vi "GetImage.vi"(0 "XRef":T4, 1 "State In":T3) -> (14 "Image":T2, 15 "Fatal Error Out":T1)   [LabVIEW 2015, in "LVJSON.lvlib" / "Build JSON Array.xnode"]
uses:
  Build JSON Array.xnode
  <vilib>/XNodeSupport/XNodeXNodeRef.ctl
  State.ctl
  <vilib>/XNodeSupport/XNodeImage.ctl
  <vilib>/XNodeSupport/XNodeErrorCluster.ctl
  dimensions.vi
  <vilib>/XNodeSupport/NI_XNodeSupport.lvlib
panel:
  out "image depth 2":i32
  out "image type 2":i32
  out "image depth":i32
  out "image type":i32
  out "size(s) 2":i32
  out "size(s)":i32
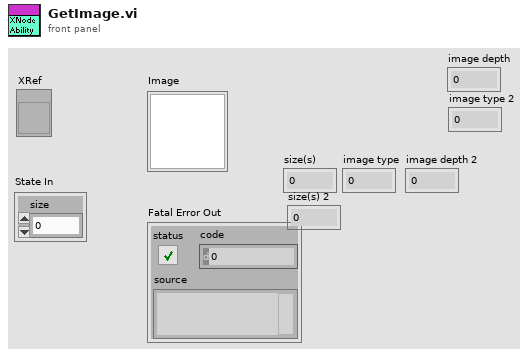
[diagram p1: front panel]
types:
  T1 = typedef "NI_XNodeSupport.lvlib/XNodeErrorCluster.ctl" = errorcluster
  T2 = typedef "NI_XNodeSupport.lvlib/XNodeImage.ctl" = picture
  T3 = typedef "LVJSON.lvlib/Build JSON Array.xnode/State.ctl" = cluster{"size":u32}
  T4 = typedef "NI_XNodeSupport.lvlib/XNodeXNodeRef.ctl" = refnum<vi>
  T5 = typedef "imagedata.ctl" = cluster{"image type":i32, "image depth":i32, "image":u8[], "mask":u8[], "colors":u32[], "Rectangle":cluster{"left":i16, "top":i16, "right":i16, "bottom":i16}}
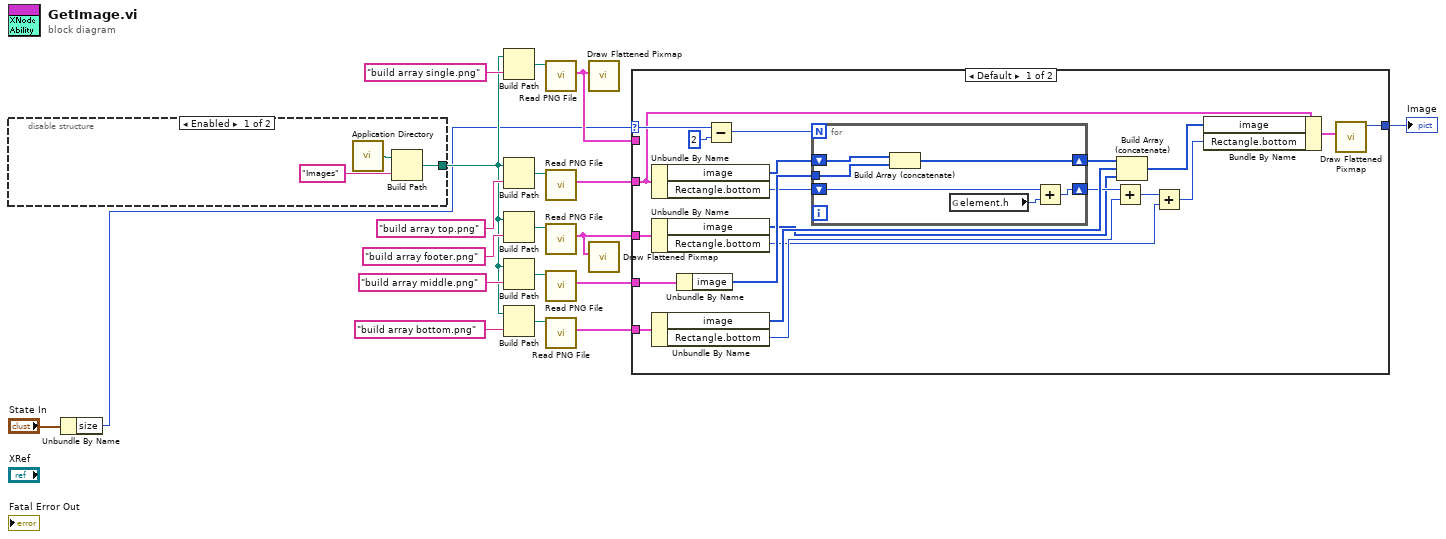
[diagram p0: block diagram]
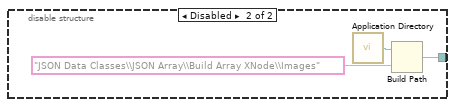
[diagram p2: hidden frame]
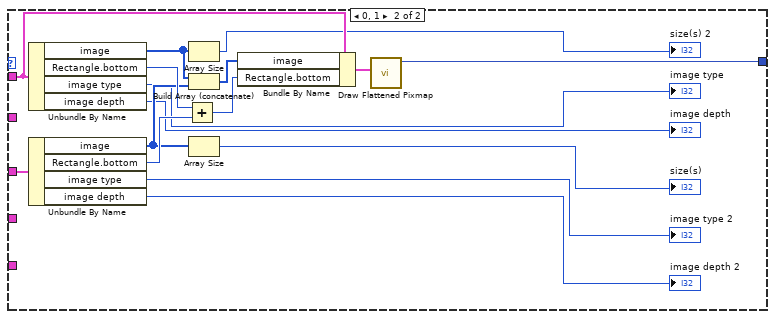
[diagram p3: hidden frame]
diagram:
  n1 = disable-structure shown="Enabled" {
    disable-tunnel: [w21 w24] -> w3
    frame Enabled {
      n2 = call <vilib>:"Application Directory.vi"() -> ("Application Directory"=w20:path)
      n3 = Build Path(base path=w20, name or relative path="Images") -> (appended path=w21:path)
    }
    frame Disabled {
      n4 = call <vilib>:"Application Directory.vi"() -> ("Application Directory"=w23:path)
      n5 = Build Path(base path=w23, name or relative path="JSON Data Classes\\JSON Array\\Build Array XNode\\Images") -> (appended path=w24:path)
    }
  }
  n6 = Unbundle By Name("State In") -> ("size"=w1:u32)
  n7 = Build Path(base path=w3, name or relative path="build array single.png") -> (appended path=w12:path)
  n8 = Build Path(base path=w3, name or relative path="build array top.png") -> (appended path=w9:path)
  n9 = Build Path(base path=w3, name or relative path="build array footer.png") -> (appended path=w5:path)
  n10 = Build Path(base path=w3, name or relative path="build array middle.png") -> (appended path=w8:path)
  n11 = Build Path(base path=w3, name or relative path="build array bottom.png") -> (appended path=w6:path)
  n12 = call <vilib>:"Read PNG File.vi"("path to PNG file"=w12) -> ("image data"=w2:T5)  [unwired: 8 in, 2 out]
  n13 = call <vilib>:"Read PNG File.vi"("path to PNG file"=w9) -> ("image data"=w17:T5)  [unwired: 8 in, 2 out]
  n14 = call <vilib>:"Read PNG File.vi"("path to PNG file"=w5) -> ("image data"=w14:T5)  [unwired: 8 in, 2 out]
  n15 = call <vilib>:"Read PNG File.vi"("path to PNG file"=w8) -> ("image data"=w16:T5)  [unwired: 8 in, 2 out]
  n16 = call <vilib>:"Read PNG File.vi"("path to PNG file"=w6) -> ("image data"=w15:T5)  [unwired: 8 in, 2 out]
  n17 = call <vilib>:"Draw Flattened Pixmap.vi"("image data"=w2) -> ()  [unwired: 8 in, 1 out]
  n18 = call <vilib>:"Draw Flattened Pixmap.vi"("image data"=w14) -> ()  [unwired: 8 in, 1 out]
  n19 = case shown="Default" w1 {
    selector: w1 -> [w45 _]
    tunnel: [w40 w68] -> w18
    tunnel: w17 -> [w33 _]
    tunnel: w16 -> [w32 _]
    tunnel: w15 -> [w31 _]
    tunnel: w2 -> [_ w66]
    tunnel: w14 -> [w29 w67]
    frame Default {
      n20 = Unbundle By Name(w33) -> ("image"=w46:u8[], "Rectangle.bottom"=w39:i16)
      n21 = Unbundle By Name(w29) -> ("image"=w28:u8[], "Rectangle.bottom"=w27:i16)
      n22 = Unbundle By Name(w31) -> ("image"=w37:u8[], "Rectangle.bottom"=w34:i16)
      n23 = Unbundle By Name(w32) -> ("image"=w42:u8[])
      n24 = Subtract(x=w45, y=2) -> (x-y=w43:u32)
      n25 = for {
        N: w43 -> [_]
        shift-right: [w50] -> w38
        shift-left: w46 -> [w52]
        tunnel: w42 -> [w51]
        shift-right: [w47] -> w35
        shift-left: w39 -> [w49]
        n26 = Build Array (concatenate)(w52, w51) -> (w50:u8[])
        n27 = global read "dimensions.vi" "element.h"() -> (w48:i16)
        n28 = Add(x=w49, y=w48) -> (x+y=w47:i16)
      }
      n29 = Add(x=w35, y=w34) -> (x+y=w30:i16)
      n30 = Build Array (concatenate)(w38, w37, w28) -> (w36:u8[])
      n31 = Add(x=w30, y=w27) -> (x+y=w26:i16)
      n32 = Bundle By Name(cluster=w33, "image"=w36, "Rectangle.bottom"=w26) -> (w41:T5)
      n33 = call <vilib>:"Draw Flattened Pixmap.vi"("image data"=w41) -> ("new picture"=w40:picture)  [unwired: 8 in]
    }
    frame 0, 1 {
      n34 = Unbundle By Name(w66) -> ("image"=w57:u8[], "Rectangle.bottom"=w64:i16, "image type"=→"image type":i32, "image depth"=→"image depth":i32)
      n35 = Unbundle By Name(w67) -> ("image"=w60:u8[], "Rectangle.bottom"=w63:i16, "image type"=→"image type 2":i32, "image depth"=→"image depth 2":i32)
      n36 = Add(x=w64, y=w63) -> (x+y=w62:i16)
      n37 = Array Size(array=w57) -> (size(s)=→"size(s) 2":i32)
      n38 = Build Array (concatenate)(w57, w60) -> (w65:u8[])
      n39 = Array Size(array=w60) -> (size(s)=→"size(s)":i32)
      n40 = Bundle By Name(cluster=w66, "image"=w65, "Rectangle.bottom"=w62) -> (w61:T5)
      n41 = call <vilib>:"Draw Flattened Pixmap.vi"("image data"=w61) -> ("new picture"=w68:picture)  [unwired: 8 in]
    }
  }
  "Image" <- w18
